vi "Configure Step Detection.vi"(8 "error in (no error)":errorcluster, 10 "Step Det":bool, 11 "PM-EMP in":refnum<class "PM-EMP.lvclass">) -> (0 "error out":errorcluster, 3 "PM-EMP out":refnum<class "PM-EMP.lvclass">)   [LabVIEW 2020, in "PM-EMP.lvclass"]
uses:
  PM-EMP.lvclass
  C:/Sandbox/RF Bench/Source Code/WiSpry Test Framework/Instruments/Instrument.lvclass
  C:/Sandbox/RF Bench/Source Code/WiSpry Test Framework/Instruments/Power Meter/Power Meter.lvclass
  Instrument.lvclass/Instrument.ctl
  Power Meter.lvclass/Power Meter.ctl
  Instrument.lvclass
  Power Meter.lvclass
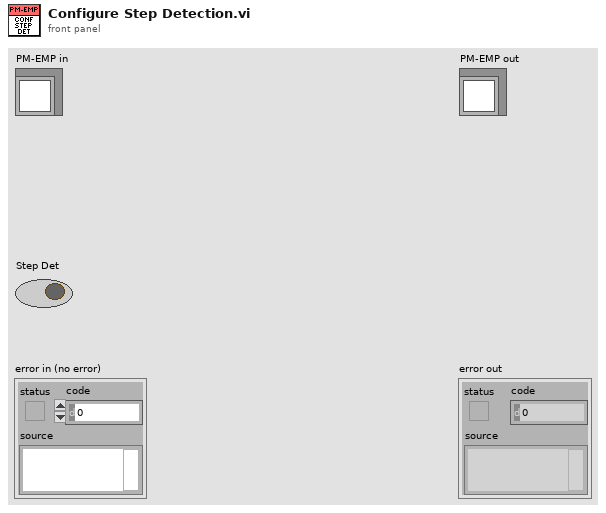
[diagram p1: front panel]
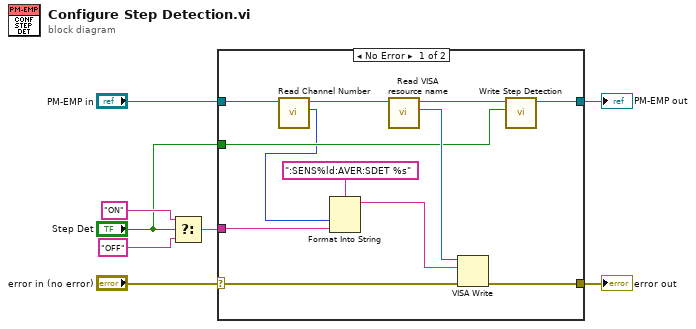
[diagram p0: block diagram]
diagram:
  n1 = Select(t="ON", s="Step Det", f="OFF") -> (s? t:f=w2:string)
  n2 = case shown="No Error" "error in (no error)" {
    selector: "error in (no error)" -> [w16 w21]
    tunnel: [w19 w21] -> w7
    tunnel: "PM-EMP in" -> [w11 w22]
    tunnel: [w13 w22] -> w5
    tunnel: w2 -> [w15 _]
    tunnel: "Step Det" -> [w12 _]
    frame No Error {
      n3 = call-dynamic "Read Channel Number.vi"("Power Meter in"=w11) -> ("Channel Number"=w9:u8, "Power Meter out"=w10:refnum<class "PM-EMP.lvclass">)  [unwired: 9 in]
      n4 = Format Into String(format string=":SENS%ld:AVER:SDET %s", w9, w15) -> (resulting string=w17:string)  [unwired: 2 in, 1 out]
      n5 = call "Read VISA resource name.vi"("Instrument in"=w10) -> ("VISA resource name"=w18:refnum<visa-resource-name>, "Instrument out"=w14:refnum<class "PM-EMP.lvclass">)  [unwired: 9 in]
      n6 = VISA Write(VISA resource name=w18, write buffer=w17, error in (no error)=w16) -> (error out=w19:errorcluster)  [unwired: 2 out]
      n7 = call "Write Step Detection.vi"("Step Detection"=w12, "Power Meter in"=w14) -> ("Power Meter out"=w13:refnum<class "PM-EMP.lvclass">)  [unwired: 9 in]
    }
    frame Error {
    }
  }
  "error out" <- w7
  "PM-EMP out" <- w5
